vi "Create XY Plot Histogram.vi"(8 "error in (no error)":errorcluster, 9 "Align Histogram Bin (F)":bool, 10 "Max Number of Bins (1E5)":i32=100000, 11 "Plot Histogram Call Parameters":T1={"XY Graph Refnum"=refnum, "Mouse Click Coords"={"Horizontal"=2147483647, "Vertical"=2147483647}, "Plot Index"=-1, "Bin Size"=nan}) -> (0 "error out":errorcluster, 3 "Histogram Statistics":dbl[](array[numeric]))   [LabVIEW 2019, in "Histogram Window.lvlib"]
uses:
  Histogram Window.lvlib
  Plot Histogram Call Parameters.ctl
  XY Graph Refnum.ctl
  <vilib>/Utility/miscctls.llb/LVPoint32TypeDef.ctl
  XY Graph Add-Ons.lvlib
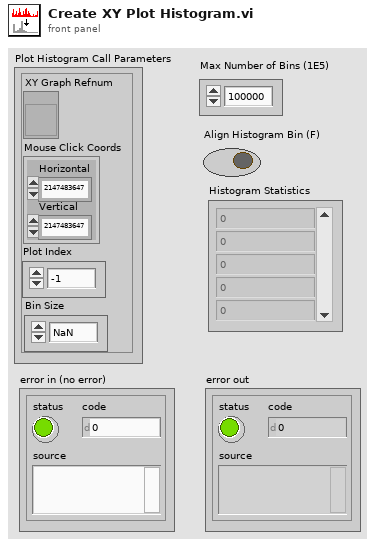
[diagram p1: front panel]
types:
  T1 = typedef "Histogram Window.lvlib/Plot Histogram Call Parameters.ctl" = cluster{"XY Graph Refnum":T2, "Mouse Click Coords":T3, "Plot Index":i32, "Bin Size":dbl}
  T2 = typedef "XY Graph Add-Ons.lvlib/XY Graph Refnum.ctl" = refnum<vi>
  T3 = typedef "LVPoint32TypeDef.ctl" = cluster{"Horizontal":i32, "Vertical":i32}
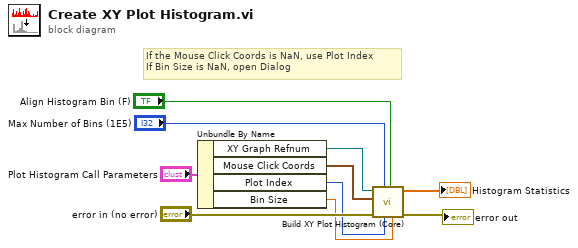
[diagram p0: block diagram]
diagram:
  # "If the Mouse Click Coords is NaN, use Plot Index\nIf Bin Size is NaN, open Dialog"
  n1 = Unbundle By Name("Plot Histogram Call Parameters") -> ("XY Graph Refnum"=w8:T2, "Mouse Click Coords"=w6:T3, "Plot Index"=w5:i32, "Bin Size"=w4:dbl)
  n2 = call "Build XY Plot Histogram (Core).vi"("Bin Size"=w4, "Align Histogram Bin"="Align Histogram Bin (F)", "Plot Index"=w5, "Max Number of Bins"="Max Number of Bins (1E5)", "error in (no error)"="error in (no error)", "Mouse Click Coords"=w6, "XYGraph in"=w8) -> ("error out"=→"error out":errorcluster, "Data Statistics"=→"Histogram Statistics":dbl[])  [unwired: 2 in, 1 out]
